vi "AutoGenerateOvenChart.vi"() -> ()   [LabVIEW 2012]
uses:
  <vilib>/addons/database/Connection.llb/DB Tools Open Connec (Path).vi
  <vilib>/addons/database/Connection.llb/Conn Execute.vi
  <vilib>/addons/database/Recordset.llb/Rec Destroy - Connection.vi
  <vilib>/addons/database/NI_Database_API.lvlib
panel:
  in  "Lot":string
  in  "Oven":string
  out "concatenated string":string
  out "error out":errorcluster
  out "array 3":string[][](array[string])
  in  "hilow":dbl=3.0
  out "array 2":string[][](array[string])
  in  "hours":dbl
  in  "target temp":dbl
  in  "Step temp":dbl
  in  "Start temp":dbl
  out "array":string[][](array[string])
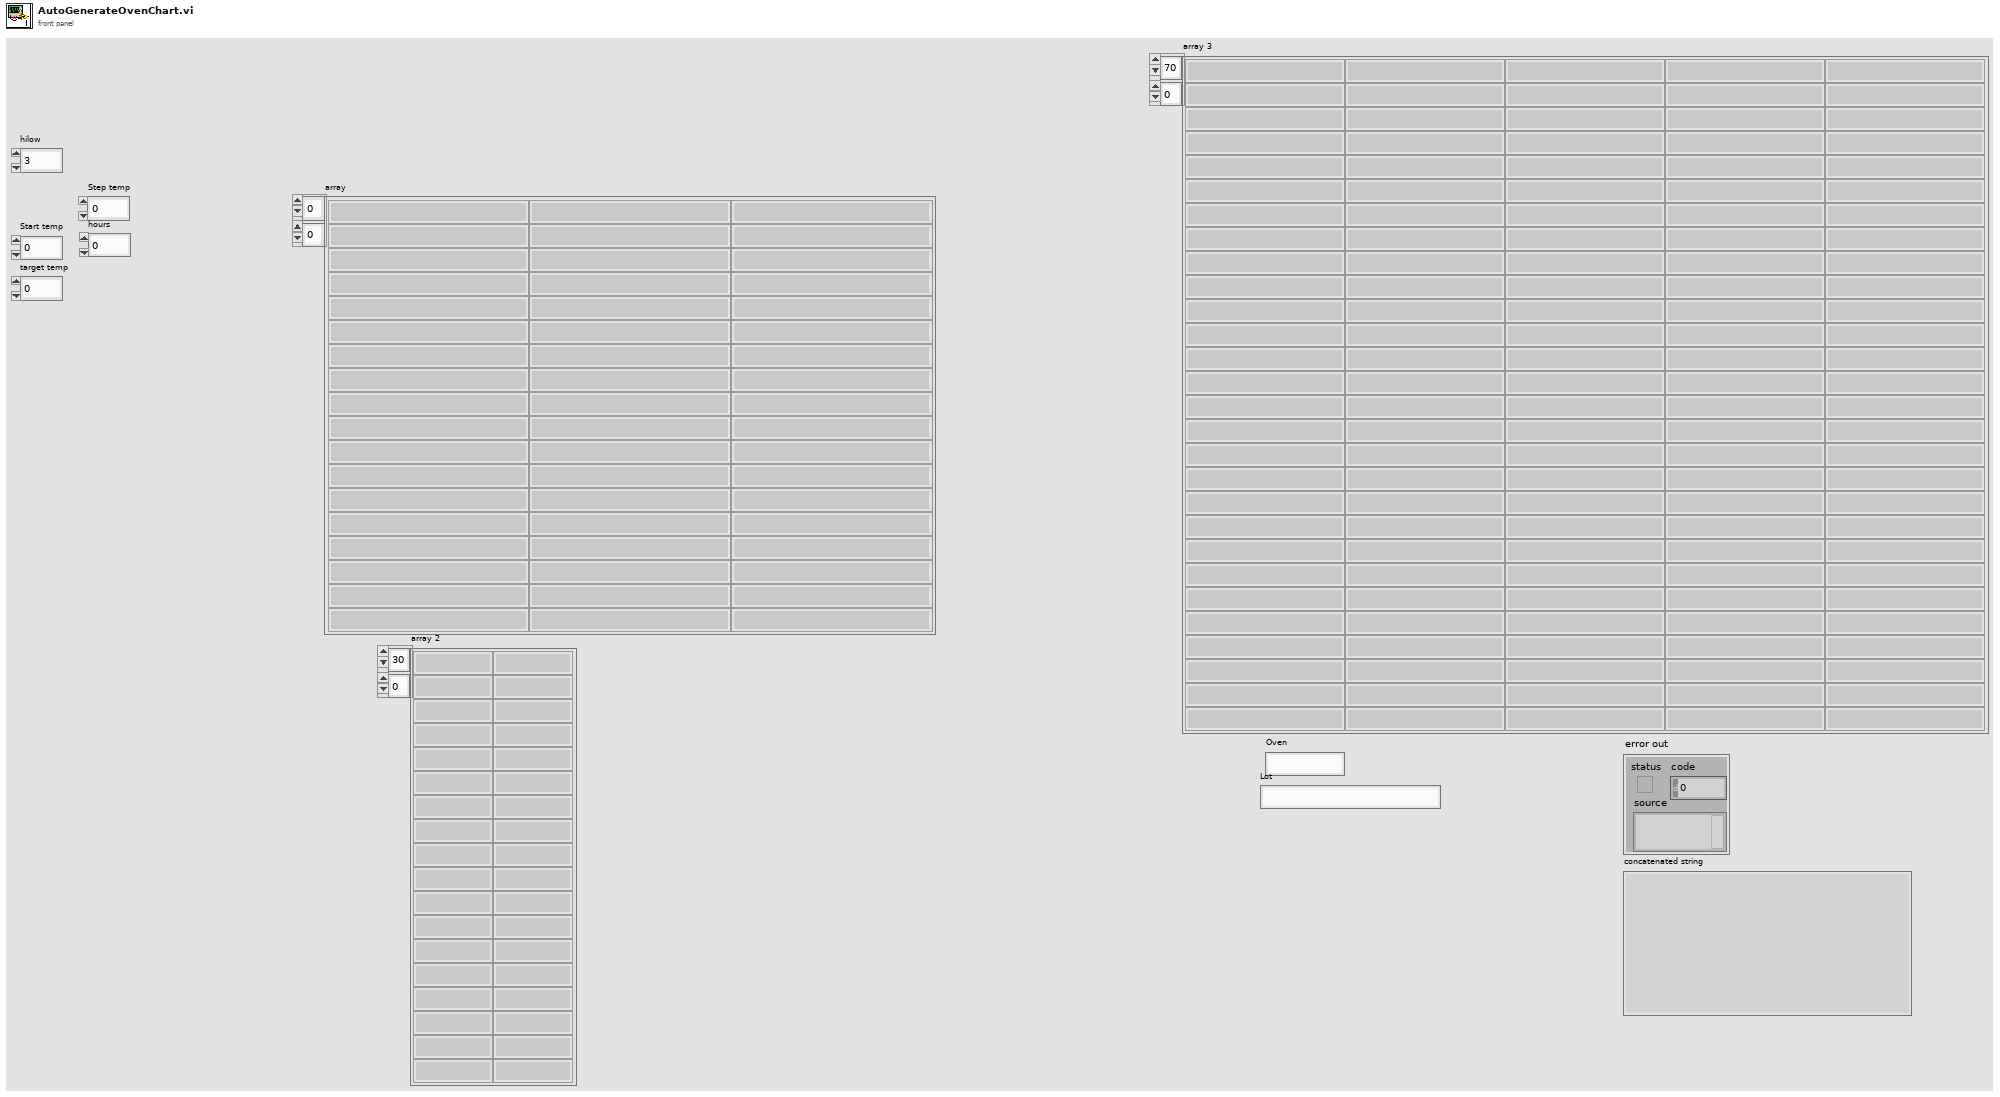
[diagram p1: front panel]
types:
  T1 = typedef "NI_Database_API.lvlib/Conn ObjectReference.ctl" = refnum<k1>
  T2 = typedef "NI_Database_API.lvlib/Rec ObjectReference.ctl" = refnum<k1>
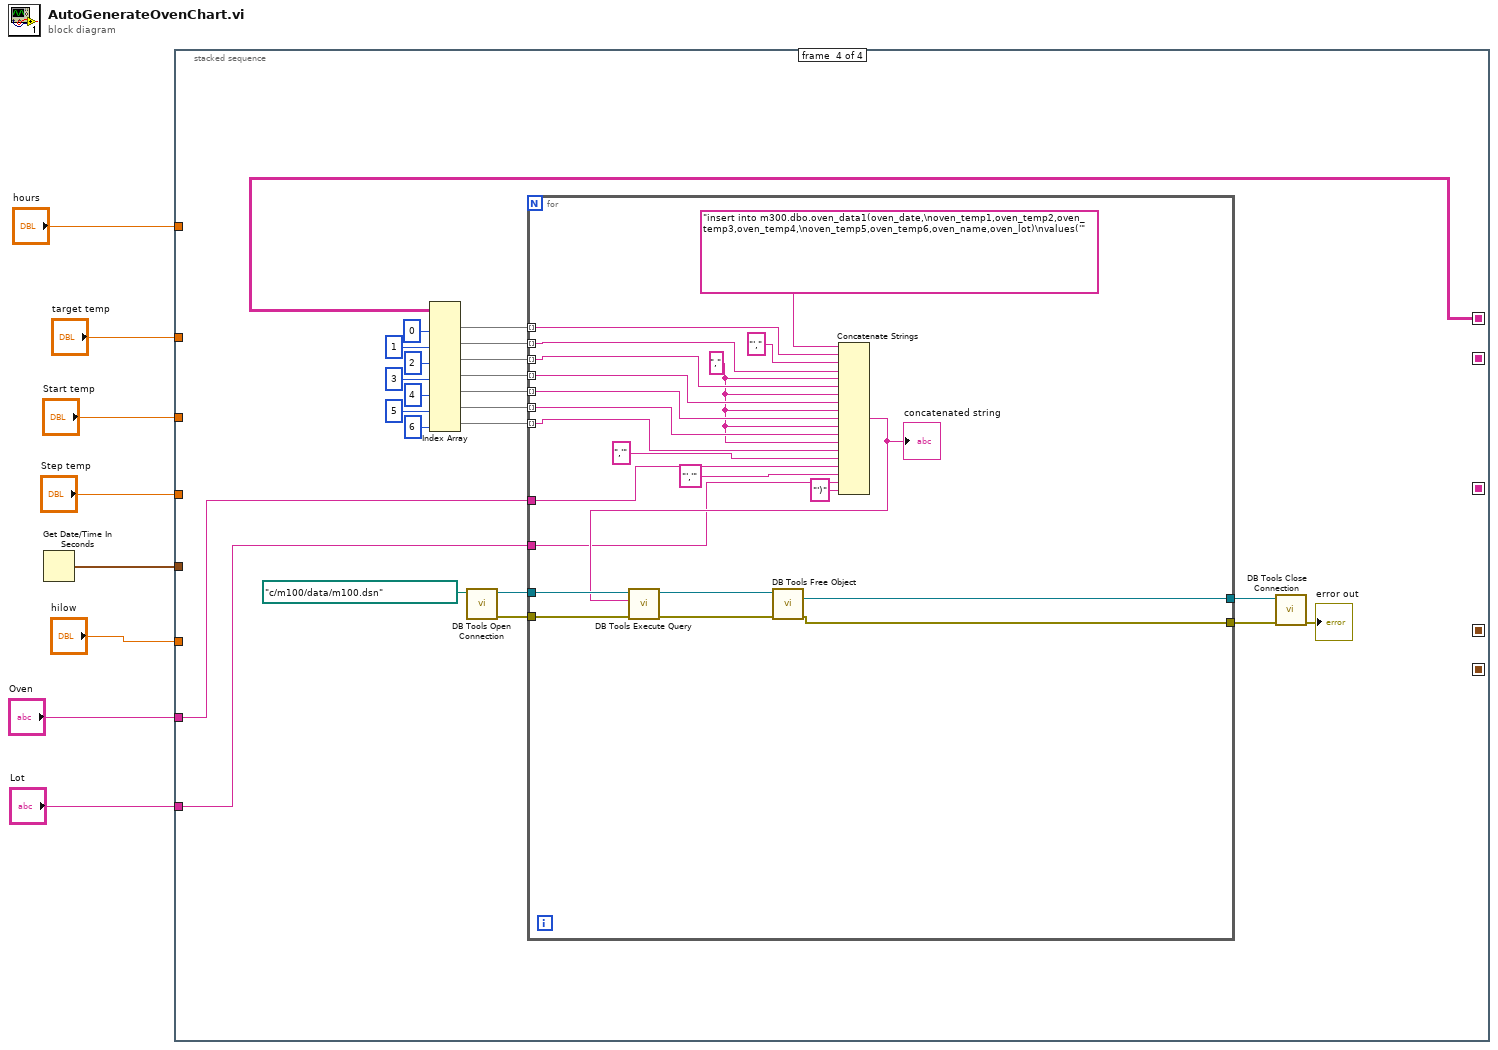
[diagram p0: block diagram]
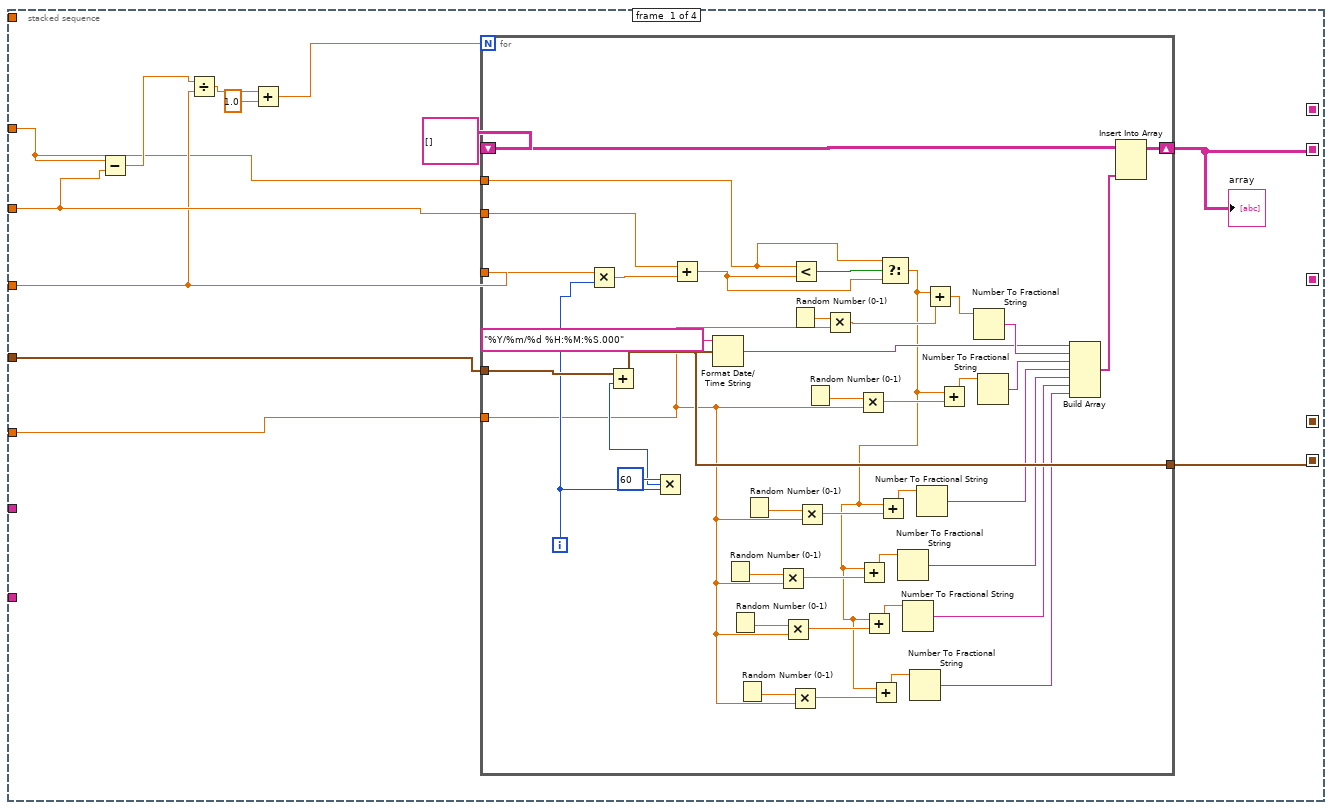
[diagram p2: hidden frame]
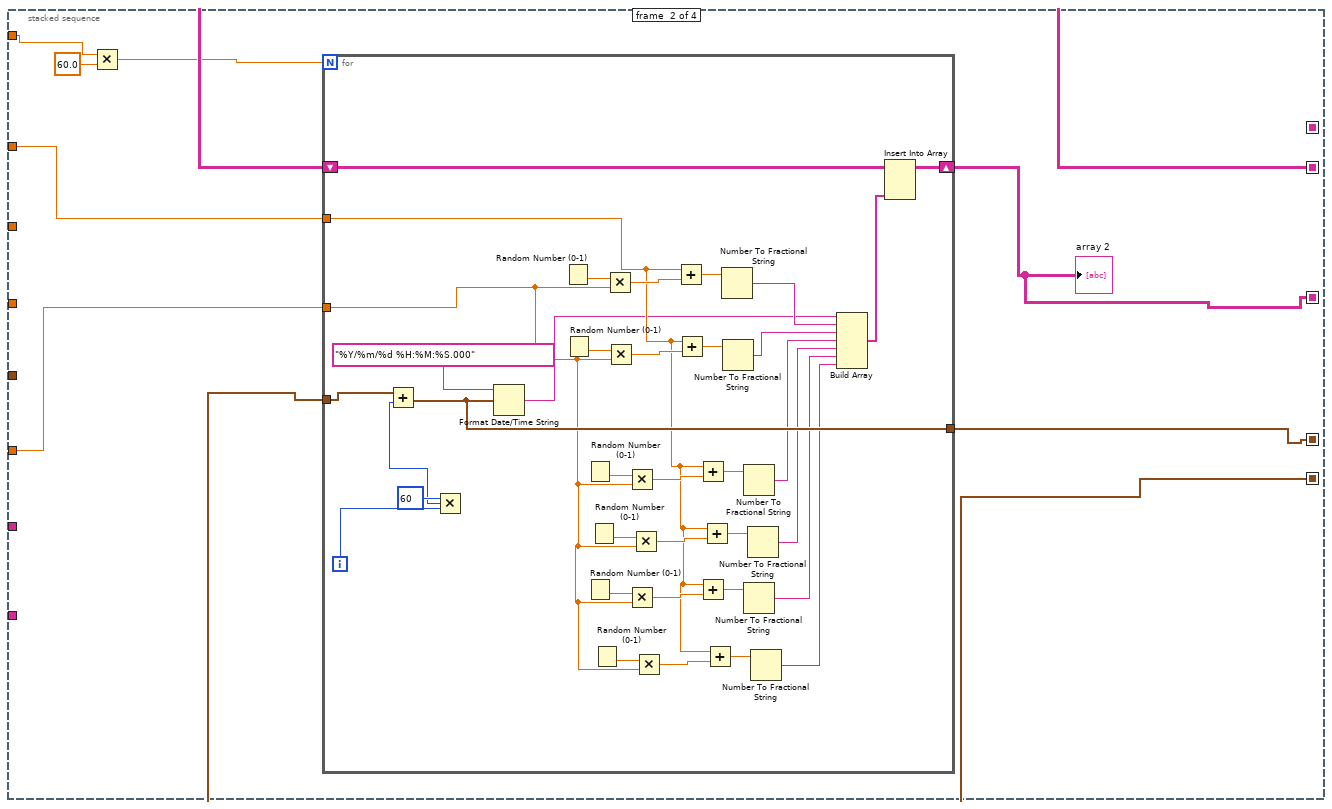
[diagram p3: hidden frame]
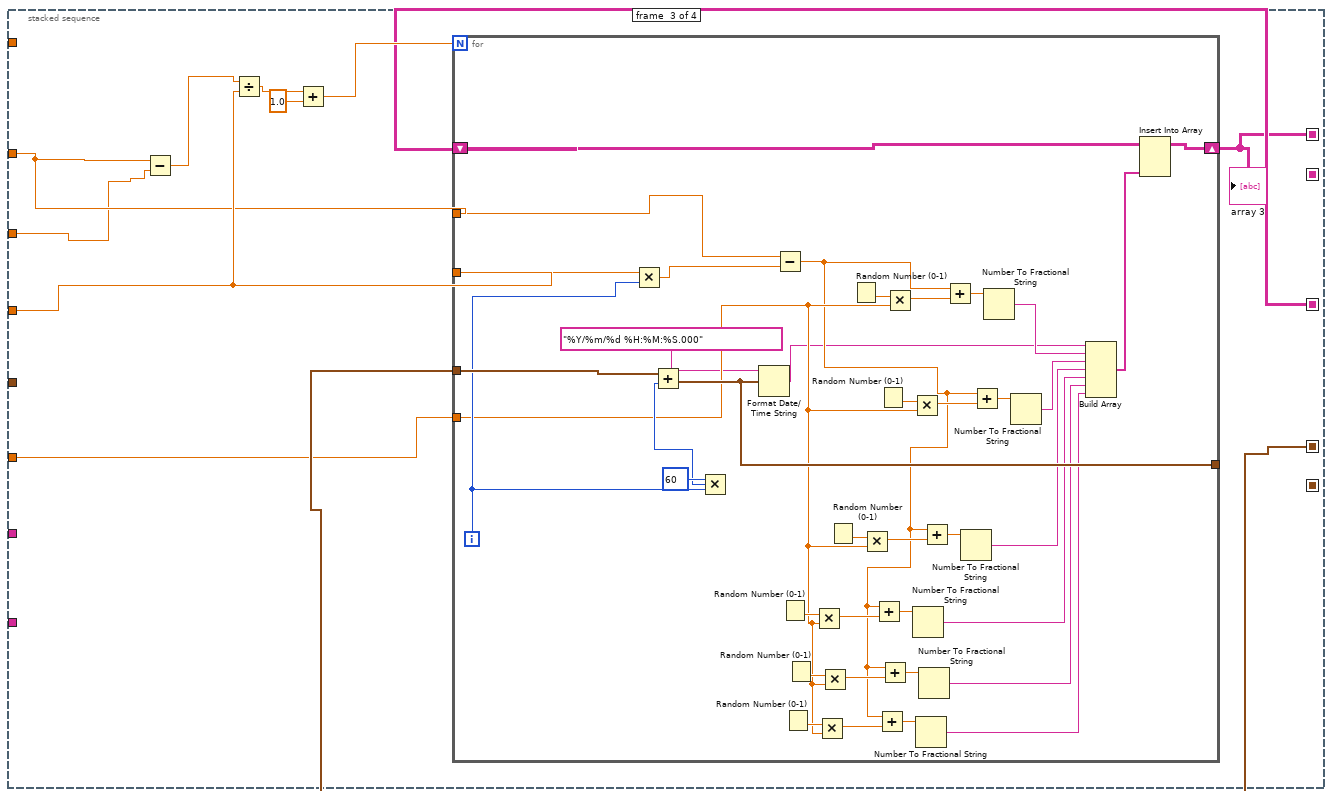
[diagram p4: hidden frame]
diagram:
  n1 = Get Date/Time In Seconds() -> (seconds since 1Jan1904=w8:timestamp)
  n2 = stacked-sequence {
    seq-local: [w9 _ _ _] -> [_ w69 _ _]
    seq-local: [w13 _ _ _] -> [_ w70 _ _]
    seq-local: [_ w64 _ _] -> [_ _ w113 _]
    seq-local: [_ w63 _ _] -> [_ _ w114 _]
    seq-local: [_ _ w108 _] -> [_ _ _ w177]
    tunnel: w8 -> [w20 _ _ _]
    tunnel: "target temp" -> [w10 w71 w110 _]
    tunnel: "Start temp" -> [w18 _ w109 _]
    tunnel: "Step temp" -> [w17 _ w111 _]
    tunnel: "hours" -> [_ w68 _ _]
    tunnel: "hilow" -> [w12 w65 w112 _]
    tunnel: "Oven" -> [_ _ _ w159]
    tunnel: "Lot" -> [_ _ _ w158]
    frame #0 {
      n3 = Subtract(x=w10, y=w18) -> (x-y=w11:dbl)
      n4 = Divide(x=w11, y=w17) -> (x/y=w16:dbl)
      n5 = Add(x=w16, y=1.0) -> (x+y=w14:dbl)
      n6 = for {
        N: w14 -> [_]
        tunnel: w20 -> [w61]
        shift-right: [w57] -> w9
        shift-left: string[][] [] ("array") -> [w56]
        tunnel: w18 -> [w55]
        tunnel: w17 -> [w54]
        tunnel: [w50] -> w13
        tunnel: w12 -> [w27]
        tunnel: w10 -> [w46]
        i -> [w53]
        n7 = Multiply(x=w54, y=w53) -> (x*y=w52:dbl)
        n8 = Multiply(x=60, y=w53) -> (x*y=w59:i32)
        n9 = Add(x=w61, y=w59) -> (x+y=w50:timestamp)
        n10 = Add(x=w55, y=w52) -> (x+y=w45:dbl)
        n11 = Format Date/Time String(time format string (%c)="%Y/%m/%d %H:%M:%S.000", seconds (now)=w50) -> (date/time string=w40:string)  [unwired: 1 in]
        n12 = Random Number (0-1)() -> (number: 0 to 1=w34:dbl)
        n13 = Random Number (0-1)() -> (number: 0 to 1=w31:dbl)
        n14 = Random Number (0-1)() -> (number: 0 to 1=w28:dbl)
        n15 = Random Number (0-1)() -> (number: 0 to 1=w37:dbl)
        n16 = Multiply(x=w34, y=w27) -> (x*y=w36:dbl)
        n17 = Multiply(x=w31, y=w27) -> (x*y=w33:dbl)
        n18 = Random Number (0-1)() -> (number: 0 to 1=w62:dbl)
        n19 = Multiply(x=w28, y=w27) -> (x*y=w30:dbl)
        n20 = Less?(x=w46, y=w45) -> (x < y?=w49:bool)
        n21 = Multiply(x=w37, y=w27) -> (x*y=w39:dbl)
        n22 = Random Number (0-1)() -> (number: 0 to 1=w42:dbl)
        n23 = Multiply(x=w62, y=w27) -> (x*y=w51:dbl)
        n24 = Multiply(x=w42, y=w27) -> (x*y=w47:dbl)
        n25 = Select(t=w46, s=w49, f=w45) -> (s? t:f=w26:dbl)
        n26 = Add(x=w26, y=w36) -> (x+y=w35:dbl)
        n27 = Add(x=w26, y=w33) -> (x+y=w32:dbl)
        n28 = Add(x=w26, y=w30) -> (x+y=w29:dbl)
        n29 = Add(x=w26, y=w39) -> (x+y=w38:dbl)
        n30 = Number To Fractional String(number=w35) -> (F-format string=w24:string)  [unwired: 3 in]
        n31 = Number To Fractional String(number=w32) -> (F-format string=w23:string)  [unwired: 3 in]
        n32 = Number To Fractional String(number=w29) -> (F-format string=w22:string)  [unwired: 3 in]
        n33 = Number To Fractional String(number=w38) -> (F-format string=w25:string)  [unwired: 3 in]
        n34 = Add(x=w26, y=w51) -> (x+y=w48:dbl)
        n35 = Add(x=w26, y=w47) -> (x+y=w44:dbl)
        n36 = Number To Fractional String(number=w48) -> (F-format string=w41:string)  [unwired: 3 in]
        n37 = Number To Fractional String(number=w44) -> (F-format string=w43:string)  [unwired: 3 in]
        n38 = Build Array(w40, w41, w43, w25, w24, w23, w22) -> (w58:string[])
        n39 = Insert Into Array(array=w56, new element=w58) -> (w57:string[][])  [unwired: 2 in]
      }
      "array" <- w9
    }
    frame #1 {
      n40 = Multiply(x=w68, y=60.0) -> (x*y=w66:dbl)
      n41 = for {
        N: w66 -> [_]
        shift-right: [w103] -> w63
        shift-left: w69 -> [w102]
        tunnel: w71 -> [w79]
        tunnel: w70 -> [w98]
        tunnel: w65 -> [w80]
        tunnel: [w97] -> w64
        i -> [w101]
        n42 = Multiply(x=60, y=w101) -> (x*y=w105:i32)
        n43 = Add(x=w98, y=w105) -> (x+y=w97:timestamp)
        n44 = Format Date/Time String(time format string (%c)="%Y/%m/%d %H:%M:%S.000", seconds (now)=w97) -> (date/time string=w73:string)  [unwired: 1 in]
        n45 = Random Number (0-1)() -> (number: 0 to 1=w107:dbl)
        n46 = Random Number (0-1)() -> (number: 0 to 1=w96:dbl)
        n47 = Random Number (0-1)() -> (number: 0 to 1=w92:dbl)
        n48 = Random Number (0-1)() -> (number: 0 to 1=w86:dbl)
        n49 = Random Number (0-1)() -> (number: 0 to 1=w89:dbl)
        n50 = Random Number (0-1)() -> (number: 0 to 1=w83:dbl)
        n51 = Multiply(x=w107, y=w80) -> (x*y=w100:dbl)
        n52 = Multiply(x=w96, y=w80) -> (x*y=w95:dbl)
        n53 = Multiply(x=w92, y=w80) -> (x*y=w91:dbl)
        n54 = Multiply(x=w86, y=w80) -> (x*y=w85:dbl)
        n55 = Multiply(x=w89, y=w80) -> (x*y=w88:dbl)
        n56 = Multiply(x=w83, y=w80) -> (x*y=w82:dbl)
        n57 = Add(x=w79, y=w100) -> (x+y=w99:dbl)
        n58 = Add(x=w79, y=w95) -> (x+y=w94:dbl)
        n59 = Add(x=w79, y=w91) -> (x+y=w90:dbl)
        n60 = Add(x=w79, y=w85) -> (x+y=w84:dbl)
        n61 = Add(x=w79, y=w88) -> (x+y=w87:dbl)
        n62 = Add(x=w79, y=w82) -> (x+y=w81:dbl)
        n63 = Number To Fractional String(number=w99) -> (F-format string=w74:string)  [unwired: 3 in]
        n64 = Number To Fractional String(number=w94) -> (F-format string=w93:string)  [unwired: 3 in]
        n65 = Number To Fractional String(number=w90) -> (F-format string=w78:string)  [unwired: 3 in]
        n66 = Number To Fractional String(number=w84) -> (F-format string=w76:string)  [unwired: 3 in]
        n67 = Number To Fractional String(number=w87) -> (F-format string=w77:string)  [unwired: 3 in]
        n68 = Number To Fractional String(number=w81) -> (F-format string=w75:string)  [unwired: 3 in]
        n69 = Build Array(w73, w74, w93, w78, w77, w76, w75) -> (w104:string[])
        n70 = Insert Into Array(array=w102, new element=w104) -> (w103:string[][])  [unwired: 2 in]
      }
      "array 2" <- w63
    }
    frame #2 {
      n71 = Subtract(x=w110, y=w109) -> (x-y=w115:dbl)
      n72 = Divide(x=w115, y=w111) -> (x/y=w118:dbl)
      n73 = Add(x=w118, y=1.0) -> (x+y=w116:dbl)
      n74 = for {
        N: w116 -> [_]
        tunnel: w113 -> [w156]
        shift-right: [w152] -> w108
        shift-left: w114 -> [w151]
        tunnel: w110 -> [w150]
        tunnel: w111 -> [w149]
        tunnel: [w145] -> _
        tunnel: w112 -> [w123]
        i -> [w148]
        n75 = Multiply(x=w149, y=w148) -> (x*y=w147:dbl)
        n76 = Multiply(x=60, y=w148) -> (x*y=w154:i32)
        n77 = Add(x=w156, y=w154) -> (x+y=w145:timestamp)
        n78 = Format Date/Time String(time format string (%c)="%Y/%m/%d %H:%M:%S.000", seconds (now)=w145) -> (date/time string=w120:string)  [unwired: 1 in]
        n79 = Subtract(x=w150, y=w147) -> (x-y=w122:dbl)
        n80 = Random Number (0-1)() -> (number: 0 to 1=w136:dbl)
        n81 = Random Number (0-1)() -> (number: 0 to 1=w130:dbl)
        n82 = Random Number (0-1)() -> (number: 0 to 1=w133:dbl)
        n83 = Multiply(x=w136, y=w123) -> (x*y=w135:dbl)
        n84 = Multiply(x=w130, y=w123) -> (x*y=w129:dbl)
        n85 = Multiply(x=w133, y=w123) -> (x*y=w132:dbl)
        n86 = Random Number (0-1)() -> (number: 0 to 1=w139:dbl)
        n87 = Random Number (0-1)() -> (number: 0 to 1=w157:dbl)
        n88 = Multiply(x=w139, y=w123) -> (x*y=w138:dbl)
        n89 = Add(x=w122, y=w135) -> (x+y=w134:dbl)
        n90 = Add(x=w122, y=w129) -> (x+y=w128:dbl)
        n91 = Random Number (0-1)() -> (number: 0 to 1=w143:dbl)
        n92 = Add(x=w122, y=w132) -> (x+y=w131:dbl)
        n93 = Multiply(x=w157, y=w123) -> (x*y=w146:dbl)
        n94 = Multiply(x=w143, y=w123) -> (x*y=w142:dbl)
        n95 = Number To Fractional String(number=w134) -> (F-format string=w126:string)  [unwired: 3 in]
        n96 = Number To Fractional String(number=w128) -> (F-format string=w124:string)  [unwired: 3 in]
        n97 = Number To Fractional String(number=w131) -> (F-format string=w125:string)  [unwired: 3 in]
        n98 = Add(x=w122, y=w138) -> (x+y=w137:dbl)
        n99 = Add(x=w122, y=w146) -> (x+y=w144:dbl)
        n100 = Number To Fractional String(number=w137) -> (F-format string=w127:string)  [unwired: 3 in]
        n101 = Add(x=w122, y=w142) -> (x+y=w141:dbl)
        n102 = Number To Fractional String(number=w144) -> (F-format string=w121:string)  [unwired: 3 in]
        n103 = Number To Fractional String(number=w141) -> (F-format string=w140:string)  [unwired: 3 in]
        n104 = Build Array(w120, w121, w140, w127, w126, w125, w124) -> (w153:string[])
        n105 = Insert Into Array(array=w151, new element=w153) -> (w152:string[][])  [unwired: 2 in]
      }
      "array 3" <- w108
    }
    frame #3 {
      n106 = Index Array(array=w177, index (col) #1=0 ("disabled index (col)"), index (col) #2=1 ("index (col)"), index (col) #3=2 ("index (col)"), index (col) #4=3 ("index (col)"), index (col) #5=4 ("index (col)"), index (col) #6=5 ("index (col)"), index (col) #7=6 ("index (col)")) -> (element #1=w169:string[], element #2=w168:string[], element #3=w167:string[], element #4=w166:string[], element #5=w165:string[], element #6=w164:string[], element #7=w163:string[])  [unwired: 7 in]
      n107 = call-poly <vilib>:"DB Tools Open Connection.vi"("connection information"=path "c:/m100/data/m100.dsn") -> ("error out"=w179:errorcluster, "connection reference"=w180:T1)  [unwired: 7 in]
      n108 = for {
        tunnel: w180 -> [w202]
        tunnel: w179 -> [w200]
        tunnel: w169 -> [w197] mode=indexing
        tunnel: w168 -> [w195] mode=indexing
        tunnel: w167 -> [w194] mode=indexing
        tunnel: w166 -> [w193] mode=indexing
        tunnel: w165 -> [w192] mode=indexing
        tunnel: w164 -> [w191] mode=indexing
        tunnel: w163 -> [w189] mode=indexing
        tunnel: [w187] -> w162
        tunnel: [w186] -> w161
        tunnel: w159 -> [w184]
        tunnel: w158 -> [w182]
        w190 = "," ("string")
        n109 = Concatenate Strings("insert into m300.dbo.oven_data1(oven_date,\noven_temp1,oven_temp2,oven_temp3,oven_temp4,\noven_temp5,oven_temp6,oven_name,oven_lot)\nvalues('" ("string"), w197, "'," ("string"), w195, w190, w194, w190, w193, w190, w192, w190, w191, w190, w189, ",'" ("string"), w184, "','" ("string"), w182, "')" ("string")) -> (w188:string)
        "concatenated string" <- w188
        n110 = call-poly <vilib>:"DB Tools Execute Query.vi"("error in (no error)"=w200, "SQL query"=w188, "connection reference"=w202) -> ("error out"=w199:errorcluster, "recordset reference"=w201:T2)  [unwired: 5 in]
        n111 = call-poly <vilib>:"DB Tools Free Object.vi"("error in (no error)"=w199, "recordset reference"=w201) -> ("error out"=w186:errorcluster, "connection reference"=w187:T1)  [unwired: 8 in]
      }
      n112 = call <vilib>:"DB Tools Close Connection.vi"("error in (no error)"=w161, "connection reference"=w162) -> ("error out"=→"error out":errorcluster)  [unwired: 5 in]
    }
  }
